vi "Alarm Handler Test.vi"   [LabVIEW 2015]
uses:
  Re-use Libraries/Minimal Actor Framework/Actors/Base Actor/Actor/Common Config.ctl
  Re-use Libraries/Minimal Actor Framework/Actors/Base Actor/Actor/Front Panel State.ctl
  Re-use Libraries/Minimal Actor Framework/Messaging/Messenger/Messenger.lvclass
  Alarm Handler/Actor/Alarm Handler Actor.lvclass
  Re-use Libraries/Utility/Utility.lvlib
  Re-use Libraries/Minimal Actor Framework/Actors/Base Actor/Actor/Actor.lvclass
types:
  T1 = typedef "Actor.lvclass/Front Panel State.ctl" = enum32{"Invalid", "Standard", "Closed", "Hidden", "Minimized", "Maximized"}
  T2 = typedef "Actor.lvclass/Common Config.ctl" = cluster{"Launch Timeout [ms]":i32, "Wait For Launch Completed":bool, "Front Panel State":T1, "Close FP On Shutdown":bool, "Response Channel":refnum<class "Messenger.lvclass">, "Sub Panel":refnum<vi>}
  T3 = typedef "Utility.lvlib/App Paths.ctl" = cluster{"App Ini File":path, "App Data Dir":path, "Config Dir":path, "App Root Dir":path}
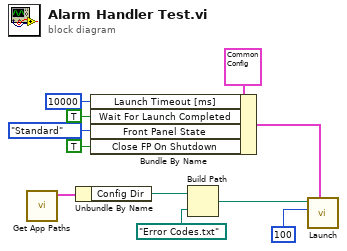
[diagram p0: block diagram]
diagram:
  n1 = call "Get App Paths.vi"() -> ("Paths"=w9:T3)  [unwired: 10 in, 1 out]
  n2 = Unbundle By Name(w9) -> ("Config Dir"=w10:path)
  n3 = Bundle By Name(cluster=T2 {"Launch Timeout [ms]"=0, "Wait For Launch Completed"=FALSE, "Front Panel State"=enum."Invalid", "Close FP On Shutdown"=FALSE, "Response Channel"=refnum, "Sub Panel"=refnum} ("Common Config"), "Launch Timeout [ms]"=10000, "Wait For Launch Completed"=TRUE ("Wait For Launch Completed (F)"), "Front Panel State"=Front_Panel_State."Standard" ("Front Panel State (Standard)"), "Close FP On Shutdown"=TRUE) -> (w5:T2)
  n4 = Build Path(base path=w10, name or relative path=path "Error Codes.txt" ("Definitions")) -> (appended path=w2:path)
  n5 = call "Launch.vi"("Common Config"=w5, "Maximum Number Of Errors"=100, "Definitions"=w2) -> ()  [unwired: 7 in, 2 out]
